vi "Sender UI.vi"(11 "error in (no error)":errorcluster) -> (15 "error out":errorcluster)   [LabVIEW 2021, in "Sender.lvclass"]
uses:
  Sender.lvclass
  Controls/Operation.ctl
  Controls/State Cluster.ctl
  Controls/Sender Data Cluster.ctl
  Controls/Communication Mode.ctl
  Communication/Communication.lvclass
  Controls/User Event Operation.ctl
  Downloads/Sample PC Template/Sample PC Template/Typedefs/Data.ctl
  Downloads/Sample PC Template/Sample PC Template/Sample PC Template.lvlib
panel:
  in  "Stop Data":bool
  in  "Transmission Type":T1
  in  "Data Type":string(combo)
  in  "Send":bool
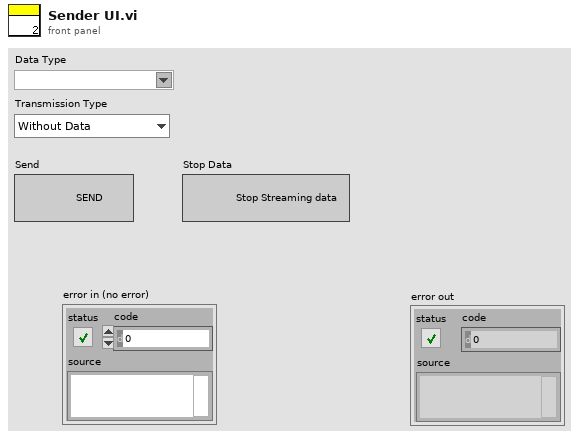
[diagram p1: front panel]
types:
  T1 = typedef "Communication Mode.ctl" = enum16{"Without Data", "With Data", "Stream Data"}
  T2 = typedef "User Event Operation.ctl" = enum16{"Obtain", "Generate", "Release"}
  T3 = typedef "Sender Data Cluster.ctl" = cluster{"user event out":refnum<user-event>, "Selected Data Type":string, "Receiver VI Reference":refnum<vi>, "Transmission Type":T1, "Start Time":dbl, "Stop Stream Data":bool}
  T4 = typedef "State Cluster.ctl" = cluster{"State":string, "Data":variant}
  T5 = typedef "Operation.ctl" = enum16{"Create", "Enqueue", "Enqueue N", "Enstack", "Dequeue", "Flush", "Release"}
  T6 = typedef "Sample PC Template.lvlib/Data.ctl" = cluster{"State":string, "Data":variant}
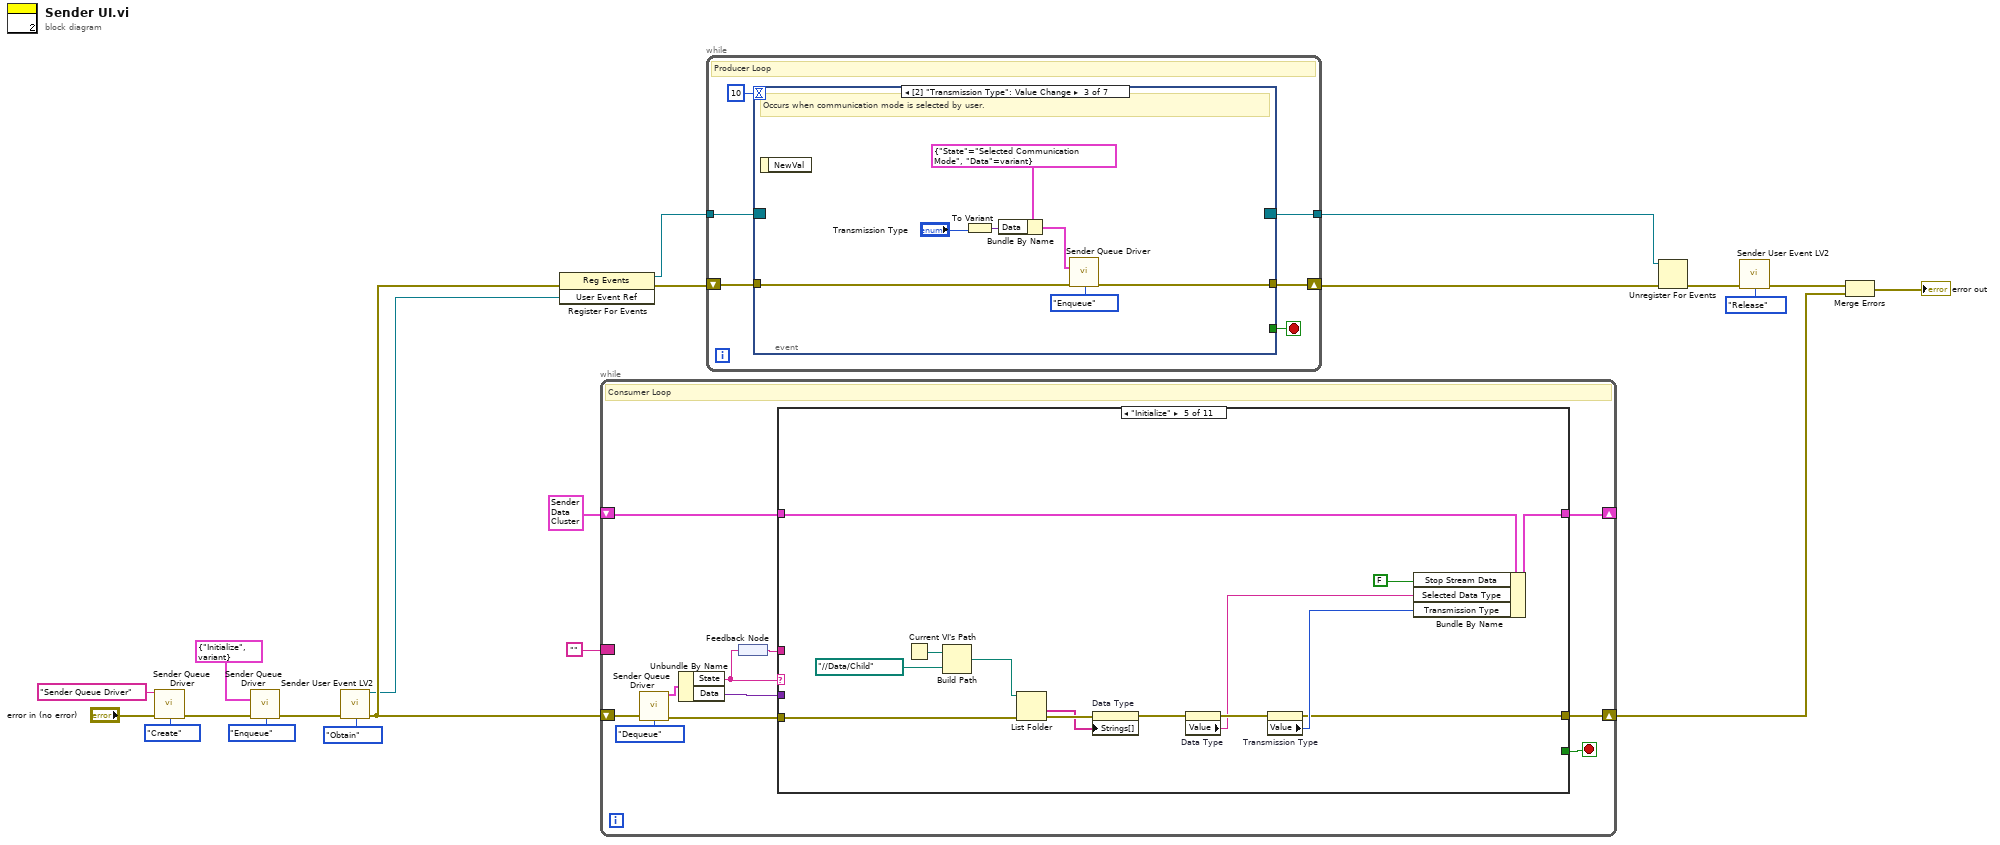
[diagram p0: block diagram]
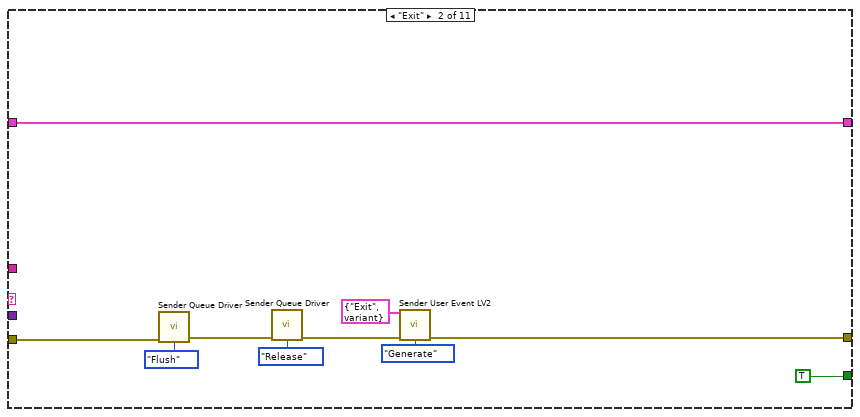
[diagram p3: hidden frame]
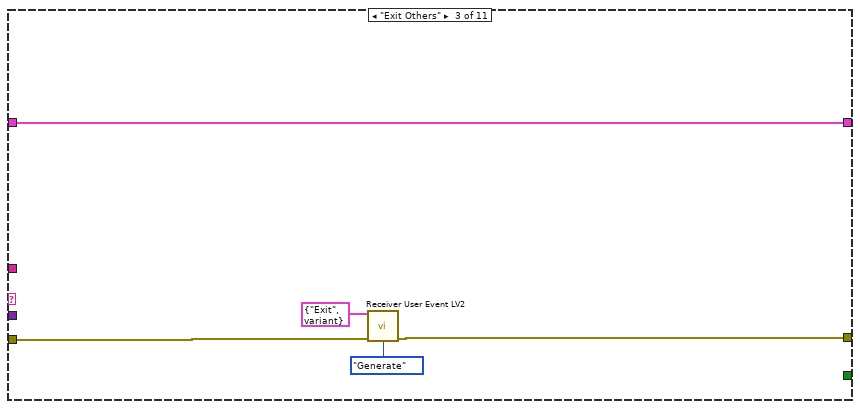
[diagram p4: hidden frame]
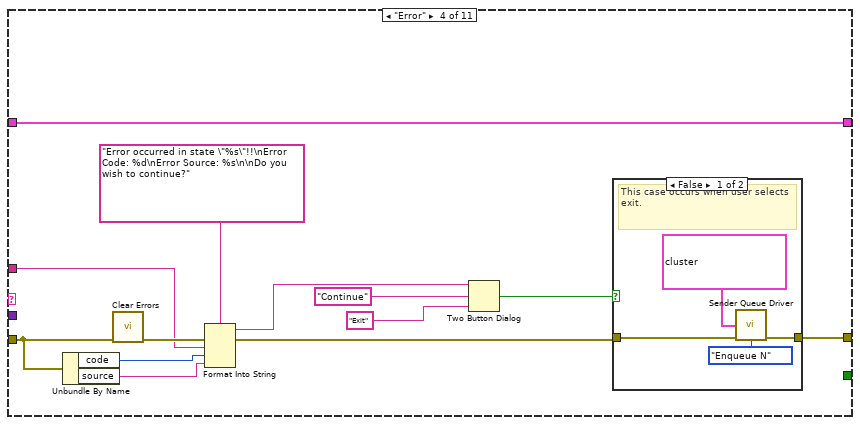
[diagram p5: hidden frame]
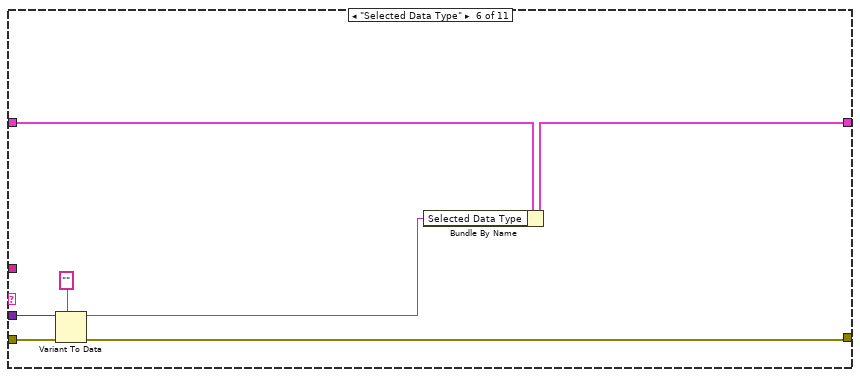
[diagram p7: hidden frame]
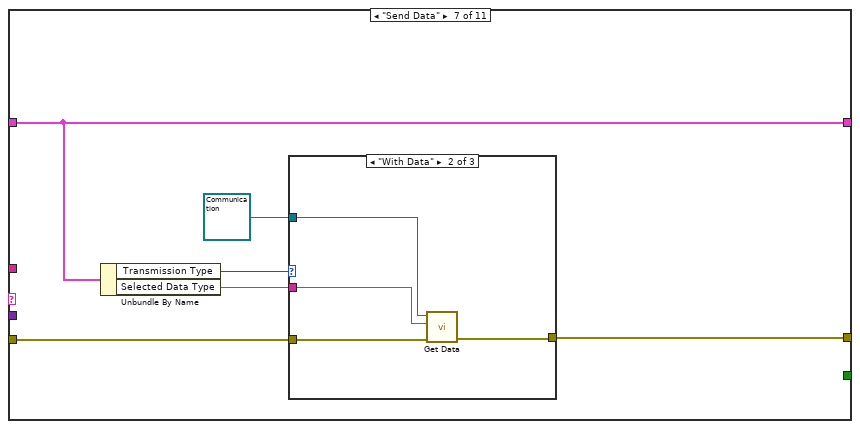
[diagram p8: hidden frame]
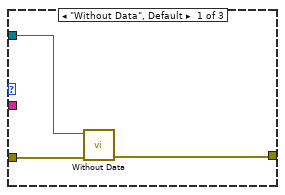
[diagram p9: hidden frame]
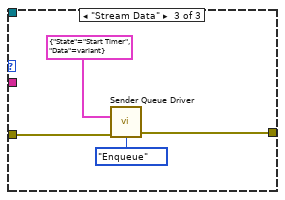
[diagram p10: hidden frame]
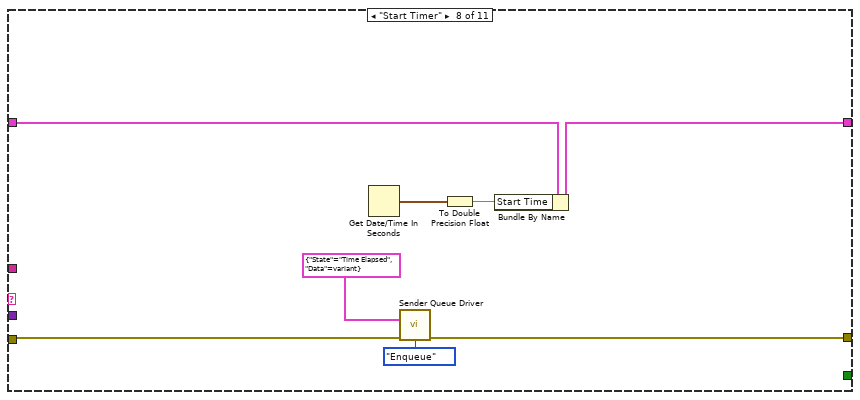
[diagram p11: hidden frame]
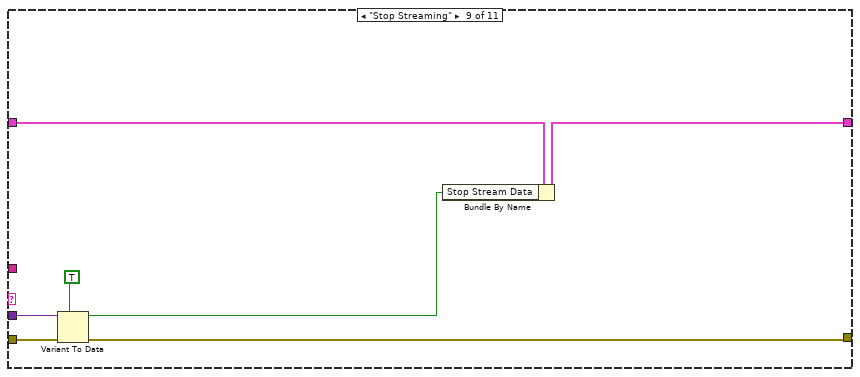
[diagram p12: hidden frame]
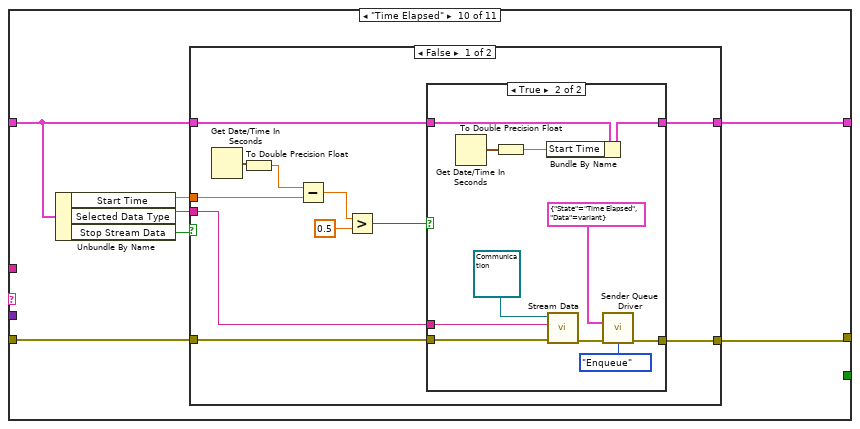
[diagram p13: hidden frame]
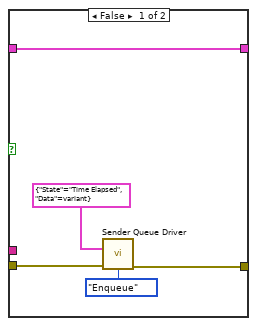
[diagram p14: hidden frame]
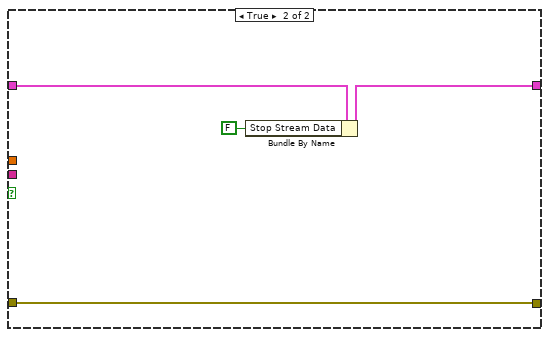
[diagram p15: hidden frame]
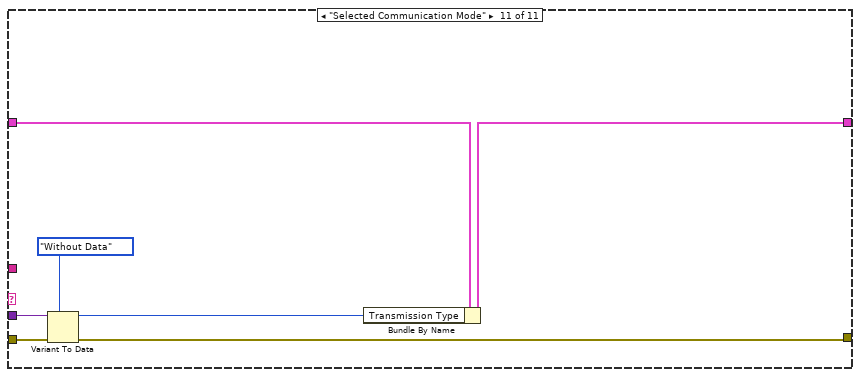
[diagram p16: hidden frame]
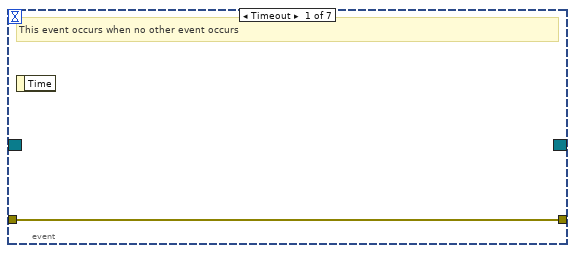
[diagram p17: hidden frame]
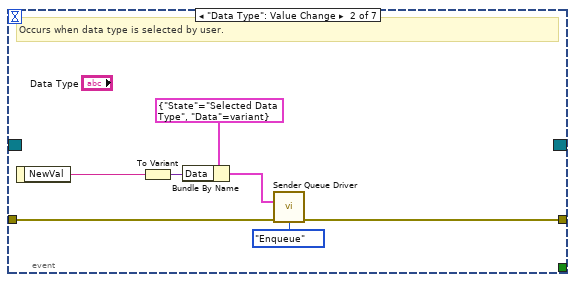
[diagram p18: hidden frame]
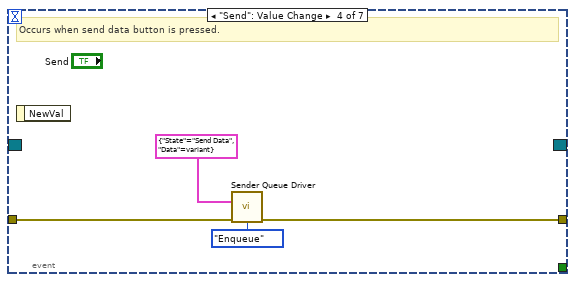
[diagram p19: hidden frame]
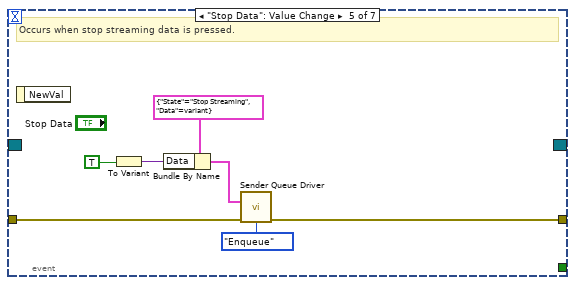
[diagram p20: hidden frame]
diagram:
  n1 = call "Sender Queue Driver.vi"("Queue Name"="Sender Queue Driver", "error in (no error)"="error in (no error)", "Operations"=Operation."Create") -> ("error out"=w19:errorcluster)  [unwired: 11 in, 1 out]
  n2 = call "Sender Queue Driver.vi"("State"=T4 {"State"="Initialize", "Data"=variant}, "error in (no error)"=w19, "Operations"=Operation."Enqueue") -> ("error out"=w7:errorcluster)  [unwired: 11 in, 1 out]
  n3 = call "Sender User Event LV2.vi"("Error In"=w7, "Operation"=User_Event_Operation."Obtain") -> ("User Event Ref"=w4:refnum<user-event>, "Error Out"=w6:errorcluster)  [unwired: 12 in]
  n4 = register-events(error in=w6, w4) -> (reference out=w13:refnum<event-registration>, error out=w14:errorcluster)  [unwired: 1 in]
  n5 = while {
    shift-right: [w25] -> w9
    shift-left: w6 -> [w31]
    border: "" -> [_]
    shift-right: [w22] -> _
    shift-left: T3 {"user event out"=refnum, "Selected Data Type"="", "Receiver VI Reference"=refnum, "Transmission Type"=enum."Without Data", "Start Time"=0.0, "Stop Stream Data"=FALSE} -> [w23]
    stop <- w24 stop-if-true
    # "Consumer Loop"
    n6 = call "Sender Queue Driver.vi"("error in (no error)"=w31, "Operations"=Operation."Dequeue") -> ("Dequeued Element"=w30:T4, "error out"=w28:errorcluster)  [unwired: 12 in]
    n7 = Unbundle By Name(w30) -> ("State"=w27:string, "Data"=w29:variant)
    n8 = feedback-in #1(w27) -> ()
    n9 = feedback #1() -> (w26:string)
    n10 = case shown="\"Initialize\"" w27 {
      tunnel: w29 -> [_ _ _ _ _ w87 _ _ w117 _ w163]
      tunnel: w28 -> [w34 w43 w48 w55 w77 w88 w94 w109 w120 w126 w165]
      tunnel: w26 -> [_ _ _ w51 _ _ _ _ _ _ _]
      tunnel: [w34 w37 w47 w54 w68 w85 w93 w108 w119 w125 w164] -> w25
      tunnel: [_ TRUE _ _ _ _ _ _ _ _ _] -> w24
      tunnel: w23 -> [w33 w39 w49 w50 w81 w84 w92 w113 w116 w123 w161]
      tunnel: [w33 w39 w49 w50 w80 w83 w92 w112 w115 w122 w159] -> w22
      frame Default {
      }
      frame "Exit" {
        n11 = call "Sender Queue Driver.vi"("error in (no error)"=w43, "Operations"=Operation."Flush") -> ("error out"=w42:errorcluster)  [unwired: 12 in, 1 out]
        n12 = call "Sender Queue Driver.vi"("error in (no error)"=w42, "Operations"=Operation."Release") -> ("error out"=w38:errorcluster)  [unwired: 12 in, 1 out]
        n13 = call "Sender User Event LV2.vi"("Data"=T6 {"State"="Exit", "Data"=variant}, "Error In"=w38, "Operation"=User_Event_Operation."Generate") -> ("Error Out"=w37:errorcluster)  [unwired: 11 in, 1 out]
      }
      frame "Exit Others" {
        n14 = call "Receiver User Event LV2.vi"("Data"=T6 {"State"="Exit", "Data"=variant}, "Error In"=w48, "Operation"=User_Event_Operation."Generate") -> ("Error Out"=w47:errorcluster)  [unwired: 11 in, 1 out]
      }
      frame "Error" {
        n15 = Unbundle By Name(w55) -> ("code"=w53:i32, "source"=w52:string)
        n16 = call <vilib>:"Clear Errors.vi"("error in (no error)"=w55) -> ("error out"=w62:errorcluster)  [unwired: 5 in, 1 out]
        n17 = Format Into String(format string="Error occurred in state \"%s\"!!\nError Code: %d\nError Source: %s\n\nDo you wish to continue?", error in=w62, w51, w53, w52) -> (resulting string=w60:string, error out=w57:errorcluster)  [unwired: 1 in]
        n18 = Two Button Dialog(message=w60, 1:"Exit" ("F button name (\"Cancel\")"), 2:"Continue" ("T button name (\"OK\")")) -> (T button?=w56:bool)
        n19 = case shown="False" w56 {
          tunnel: w57 -> [w64 w67]
          tunnel: [w66 w67] -> w54
          frame False {
            # "This case occurs when user selects exit."
            n20 = call "Sender Queue Driver.vi"("State []"=T4[] [{"State"="Exit Others", "Data"=variant}, {"State"="Exit", "Data"=variant}], "error in (no error)"=w64, "Operations"=Operation."Enqueue N") -> ("error out"=w66:errorcluster)  [unwired: 11 in, 1 out]
          }
          frame True {
            # "This case occurs when user selects to continue."
          }
        }
      }
      frame "Initialize" {
        n21 = Current VI's Path() -> (path=w79:path)
        n22 = Build Path(base path=w79, name or relative path=path "../../Data/Child") -> (appended path=w76:path)
        n23 = List Folder(path=w76, error in=w77) -> (folder names=w74:string[], error out=w75:errorcluster)  [unwired: 2 in, 2 out]
        n24 = property on="Data Type" class="CmbBox"(error in=w75, "Strings[]"=w74) -> (error out=w72:errorcluster)  [unwired: 1 in, 1 out]
        n25 = property on="Data Type" class="CmbBox"(error in=w72) -> (error out=w71:errorcluster, "Value"=w69:string)  [unwired: 1 in, 1 out]
        n26 = property on="Transmission Type" class="Enum (strict)"(error in=w71) -> (error out=w68:errorcluster, "Value"=w70:T1)  [unwired: 1 in, 1 out]
        n27 = Bundle By Name(cluster=w81, "Stop Stream Data"=FALSE, "Selected Data Type"=w69, "Transmission Type"=w70) -> (w80:T3)
      }
      frame "Selected Data Type" {
        n28 = Variant To Data(error in=w88, type="", Variant=w87) -> (data=w82:string, error out=w85:errorcluster)
        n29 = Bundle By Name(cluster=w84, "Selected Data Type"=w82) -> (w83:T3)
      }
      frame "Send Data" {
        n30 = Unbundle By Name(w92) -> ("Transmission Type"=w91:T1, "Selected Data Type"=w90:string)
        n31 = case shown="\"With Data\"" w91 {
          tunnel: w94 -> [w97 w101 w105]
          tunnel: [w95 w100 w104] -> w93
          tunnel: w90 -> [_ w99 _]
          tunnel: refnum<class "Communication.lvclass"> refnum ("Communication.lvclass") -> [w96 w98 _]
          frame "Without Data", Default {
            n32 = call "Without Data.vi"("error in (no error)"=w97, "Communication in"=w96) -> ("error out"=w95:errorcluster)  [unwired: 8 in, 1 out]
          }
          frame "With Data" {
            n33 = call "Get Data.vi"("error in (no error)"=w101, "Data Type"=w99, "Communication in"=w98) -> ("error out"=w100:errorcluster)  [unwired: 7 in, 1 out]
          }
          frame "Stream Data" {
            n34 = call "Sender Queue Driver.vi"("State"=T4 {"State"="Start Timer", "Data"=variant}, "error in (no error)"=w105, "Operations"=Operation."Enqueue") -> ("error out"=w104:errorcluster)  [unwired: 11 in, 1 out]
          }
        }
      }
      frame "Start Timer" {
        n35 = Get Date/Time In Seconds() -> (seconds since 1Jan1904=w110:timestamp)
        n36 = call "Sender Queue Driver.vi"("State"=T4 {"State"="Time Elapsed", "Data"=variant}, "error in (no error)"=w109, "Operations"=Operation."Enqueue") -> ("error out"=w108:errorcluster)  [unwired: 11 in, 1 out]
        n37 = To Double Precision Float(number=w110) -> (double precision float=w111:dbl)
        n38 = Bundle By Name(cluster=w113, "Start Time"=w111) -> (w112:T3)
      }
      frame "Stop Streaming" {
        n39 = Variant To Data(error in=w120, type=TRUE, Variant=w117) -> (data=w114:bool, error out=w119:errorcluster)
        n40 = Bundle By Name(cluster=w116, "Stop Stream Data"=w114) -> (w115:T3)
      }
      frame "Time Elapsed" {
        n41 = Unbundle By Name(w123) -> ("Start Time"=w127:dbl, "Selected Data Type"=w124:string, "Stop Stream Data"=w121:bool)
        n42 = case shown="False" w121 {
          tunnel: w127 -> [w128 _]
          tunnel: w126 -> [w135 w158]
          tunnel: [w134 w158] -> w125
          tunnel: w124 -> [w132 _]
          tunnel: w123 -> [w131 w157]
          tunnel: [w130 w155] -> w122
          frame False {
            n43 = Get Date/Time In Seconds() -> (seconds since 1Jan1904=w138:timestamp)
            n44 = To Double Precision Float(number=w138) -> (double precision float=w129:dbl)
            n45 = Subtract(x=w129, y=w128) -> (x-y=w137:dbl)
            n46 = Greater?(x=w137, y=0.5) -> (0:w133:bool)
            n47 = case shown="True" w133 {
              tunnel: w135 -> [w143 w154]
              tunnel: [w142 w146] -> w134
              tunnel: w132 -> [_ w152]
              tunnel: w131 -> [w139 w151]
              tunnel: [w139 w150] -> w130
              frame False {
                n48 = call "Sender Queue Driver.vi"("State"=T4 {"State"="Time Elapsed", "Data"=variant}, "error in (no error)"=w143, "Operations"=Operation."Enqueue") -> ("error out"=w142:errorcluster)  [unwired: 11 in, 1 out]
              }
              frame True {
                n49 = Get Date/Time In Seconds() -> (seconds since 1Jan1904=w149:timestamp)
                n50 = To Double Precision Float(number=w149) -> (double precision float=w148:dbl)
                n51 = Bundle By Name(cluster=w151, "Start Time"=w148) -> (w150:T3)
                n52 = call "Stream Data.vi"("error in (no error)"=w154, "Data Type"=w152, "Communication in"=refnum<class "Communication.lvclass"> refnum ("Communication.lvclass")) -> ("error out"=w147:errorcluster)  [unwired: 7 in, 1 out]
                n53 = call "Sender Queue Driver.vi"("State"=T4 {"State"="Time Elapsed", "Data"=variant}, "error in (no error)"=w147, "Operations"=Operation."Enqueue") -> ("error out"=w146:errorcluster)  [unwired: 11 in, 1 out]
              }
            }
          }
          frame True {
            n54 = Bundle By Name(cluster=w157, "Stop Stream Data"=FALSE) -> (w155:T3)
          }
        }
      }
      frame "Selected Communication Mode" {
        n55 = Variant To Data(error in=w165, type=Communication_Mode."Without Data" ("Communication Mode"), Variant=w163) -> (data=w160:T1, error out=w164:errorcluster)
        n56 = Bundle By Name(cluster=w161, "Transmission Type"=w160) -> (w159:T3)
      }
    }
  }
  n57 = while {
    shift-right: [w168] -> w11
    shift-left: w14 -> [w169]
    tunnel: w13 -> [w170]
    tunnel: [w166] -> w10
    stop <- w167 stop-if-true
    # "Producer Loop"
    n58 = event shown="[2] \"Transmission Type\": Value Change" {
      selector: w170 -> [_ _ _ _ _ _ _]
      dyn-events: [_ _ _ _ _ _ _] -> w166
      timeout: 10 -> [_ _ _ _ _ _ _]
      tunnel: w169 -> [w172 w179 w186 w190 w197 w200 w212]
      tunnel: [w172 w178 w185 w189 w196 w198 w211] -> w168
      tunnel: [_ _ _ _ _ w199 _] -> w167
      event Timeout {
        # "This event occurs when no other event occurs"
        n59 = event-data() -> ()  [unwired: 1 in, 1 out]
      }
      event "Data Type": Value Change {
        # "Occurs when data type is selected by user."
        n60 = event-data() -> ("NewVal"=w174:string)  [unwired: 1 in]
        n61 = To Variant(anything=w174) -> (Variant=w175:variant)
        n62 = Bundle By Name(cluster=T4 {"State"="Selected Data Type", "Data"=variant} ("State"), "Data"=w175) -> (w173:T4)
        n63 = call "Sender Queue Driver.vi"("State"=w173, "error in (no error)"=w179, "Operations"=Operation."Enqueue") -> ("error out"=w178:errorcluster)  [unwired: 11 in, 1 out]
      }
      event Value Change {
        # "Occurs when communication mode is selected by user."
        n64 = event-data() -> ()  [unwired: 1 in, 1 out]
        n65 = To Variant(anything="Transmission Type") -> (Variant=w181:variant)
        n66 = Bundle By Name(cluster=T4 {"State"="Selected Communication Mode", "Data"=variant} ("State"), "Data"=w181) -> (w180:T4)
        n67 = call "Sender Queue Driver.vi"("State"=w180, "error in (no error)"=w186, "Operations"=Operation."Enqueue") -> ("error out"=w185:errorcluster)  [unwired: 11 in, 1 out]
      }
      event "Send": Value Change {
        # "Occurs when send data button is pressed."
        n68 = event-data() -> ()  [unwired: 1 in, 1 out]
        n69 = call "Sender Queue Driver.vi"("State"=T4 {"State"="Send Data", "Data"=variant}, "error in (no error)"=w190, "Operations"=Operation."Enqueue") -> ("error out"=w189:errorcluster)  [unwired: 11 in, 1 out]
      }
      event "Stop Data": Value Change {
        # "Occurs when stop streaming data is pressed."
        n70 = event-data() -> ()  [unwired: 1 in, 1 out]
        n71 = To Variant(anything=TRUE) -> (Variant=w193:variant)
        n72 = Bundle By Name(cluster=T4 {"State"="Stop Streaming", "Data"=variant} ("State"), "Data"=w193) -> (w191:T4)
        n73 = call "Sender Queue Driver.vi"("State"=w191, "error in (no error)"=w197, "Operations"=Operation."Enqueue") -> ("error out"=w196:errorcluster)  [unwired: 11 in, 1 out]
      }
      event User Event {
        n74 = event-data() -> ("State"=w201:string)  [unwired: 1 in, 1 out]
        n75 = case shown="\"Exit Consumer\"" w201 {
          tunnel: w200 -> [w202 w203 w208]
          tunnel: [_ TRUE ("Discard?") _] -> w199
          tunnel: [w202 w203 w207] -> w198
          frame Default {
          }
          frame "Exit" {
          }
          frame "Exit Consumer" {
            n76 = call "Sender Queue Driver.vi"("State"=T4 {"State"="Exit", "Data"=variant}, "error in (no error)"=w208, "Operations"=Operation."Enqueue") -> ("error out"=w207:errorcluster)  [unwired: 11 in, 1 out]
          }
        }
      }
      event Panel Close? {
        # "Occurs when panel close is pressed"
        n77 = event-data() -> ()  [unwired: 1 in, 1 out]
        n78 = call "Sender Queue Driver.vi"("State []"=T4[] [{"State"="Exit Others", "Data"=variant}, {"State"="Exit", "Data"=variant}], "error in (no error)"=w212, "Operations"=Operation."Enqueue N") -> ("error out"=w211:errorcluster)  [unwired: 11 in, 1 out]
        n79 = event-data("Discard?"=TRUE) -> ()  [unwired: 1 in, 1 out]
      }
    }
  }
  n80 = Unregister For Events(event registration refnum=w10, error in=w11) -> (error out=w3:errorcluster)
  n81 = call "Sender User Event LV2.vi"("Error In"=w3, "Operation"=User_Event_Operation."Release") -> ("Error Out"=w2:errorcluster)  [unwired: 12 in, 1 out]
  n82 = Merge Errors(w2, w9) -> (→"error out":errorcluster)
